vi "Subtract CCD thermal background.vi"(10 "Subtract CCD thermal background":bool) -> (2 "background":dbl)   [LabVIEW 2009]
uses:
  <vilib>/Utility/file.llb/Read From Spreadsheet File (DBL).vi
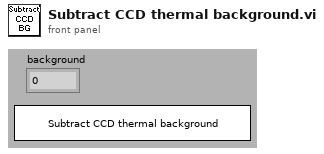
[diagram p1: front panel]
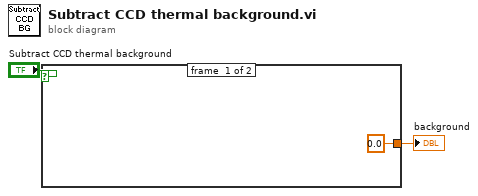
[diagram p0: block diagram]
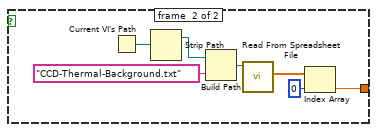
[diagram p2: hidden frame]
diagram:
  n1 = case shown="True" "Subtract CCD thermal background" {
    tunnel: [0.0 w4] -> w1
    frame #0 {
    }
    frame #1 {
      n2 = Current VI's Path() -> (path=w10:path)
      n3 = Strip Path(path=w10) -> (stripped path=w9:path)  [unwired: 1 out]
      n4 = Build Path(base path=w9, name or relative path="CCD-Thermal-Background.txt") -> (appended path=w7:path)
      n5 = call-poly <vilib>:"Read From Spreadsheet File.vi"("file path (dialog if empty)"=w7) -> ("first row"=w6:dbl[])  [unwired: 6 in, 4 out]
      n6 = Index Array(array=w6, index=0) -> (element=w4:dbl)
    }
  }
  "background" <- w1
